vi "Begin.vi"(8 "error in (no error)":errorcluster, 11 "Catapult in":refnum<class "Catapult.lvclass">) -> (0 "error out":errorcluster, 3 "Catapult out":refnum<class "Catapult.lvclass">)   [LabVIEW 2013, in "Catapult.lvclass"]
uses:
  Catapult.lvclass
  <vilib>/Rock Robotics/WPI/CAN/Jaguar/SubVIs/WPI_CANJaguar_ControlMode.ctl
  <vilib>/Rock Robotics/SystemInterfaces/Typedef/FPGA_TypedefDigitalModule.ctl
  <vilib>/Rock Robotics/SystemInterfaces/DIO/FPGA_DIOChannel.ctl
  <vilib>/Rock Robotics/WPI/Solenoid/WPI_SolenoidChannel.ctl
  <vilib>/Rock Robotics/SystemInterfaces/Typedef/FPGA_TypedefSolenoidModule.ctl
  System/System.lvclass
  <vilib>/Rock Robotics/WPI/MotorControl/WPI_MotorControlOpenCANJaguar.vi
  <vilib>/Rock Robotics/WPI/Solenoid/WPI_SolenoidOpenSingle.vi
panel:
  in  "Solenoid Module (Module 1)":T1
  in  "Solenoid Channel":T2=enum."Solenoid 2"
  in  "DIO Channel":T3=enum."DIO 2"
  in  "Digital Module (Module 1)":T4
  in  "Catapult Control Mode":T5
  in  "Catapult Device Number":u8=8
  in  "Invert Catapult Motor":bool=TRUE
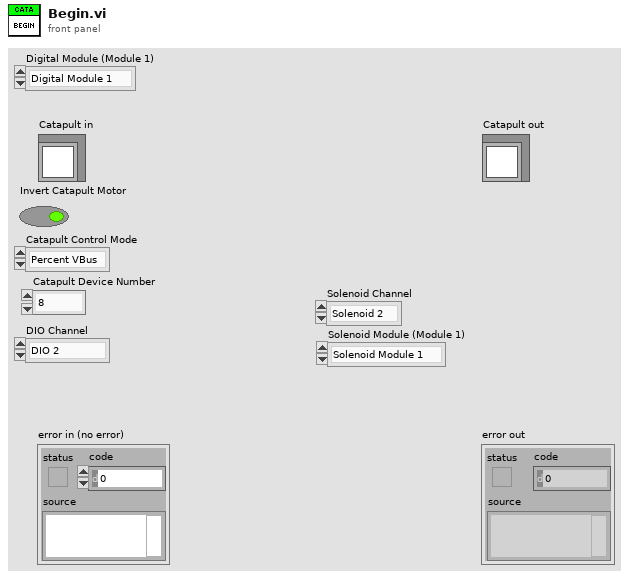
[diagram p1: front panel]
types:
  T1 = typedef "FPGA_TypedefSolenoidModule.ctl" = enum16{"Solenoid Module 1", "Solenoid Module 2"}
  T2 = typedef "WPI_SolenoidChannel.ctl" = enum8{"Solenoid 1", "Solenoid 2", "Solenoid 3", "Solenoid 4", "Solenoid 5", "Solenoid 6", "Solenoid 7", "Solenoid 8", "Invalid"}
  T3 = typedef "FPGA_DIOChannel.ctl" = enum8{"DIO 1", "DIO 2", "DIO 3", "DIO 4", "DIO 5", "DIO 6", "DIO 7", "DIO 8", "DIO 9", "DIO 10", "DIO 11", "DIO 12", "DIO 13", "DIO 14", "Invalid"}
  T4 = typedef "FPGA_TypedefDigitalModule.ctl" = enum16{"Digital Module 1", "Digital Module 2"}
  T5 = typedef "WPI_CANJaguar_ControlMode.ctl" = enum8{"Percent VBus", "Current", "Speed", "Position", "Voltage"}
  T6 = typedef "WPI_MotorControlDeviceRef.ctl" = cluster{"DeviceStatus":errorcluster, "Type":enum16{"PWM", "CAN"}, "PWM":cluster{"Digital Module":T4, "PWM Channel":T7, "DeadBand":T8}, "CAN":cluster{"Device Number":u8, "Control Mode":T5, "Semaphore":T9, "Max Vout":dbl}, "Invert":bool, "TransformRef":T10, "InvTransformRef":T10}
  T7 = typedef "FPGA_DIOPWMChannel.ctl" = enum8{"PWM 1", "PWM 2", "PWM 3", "PWM 4", "PWM 5", "PWM 6", "PWM 7", "PWM 8", "PWM 9", "PWM 10", "Invalid"}
  T8 = typedef "WPI_PWMDeadband.ctl" = cluster{"Name":string, "maxPositivePwm":i32, "minPositivePwm":i32, "centerPwm":i32, "maxNegativePwm":i32, "minNegativePwm":i32, "angularRange":u16}
  T9 = typedef "Semaphore RefNum" = refnum<k1>
  T10 = typedef "WPI_PWMTransform_ConPane.ctl" = refnum<vi>
  T11 = typedef "WPI_DigitalInputDevRef.ctl" = cluster{"DevStatus":errorcluster, "DIO Channel":T3, "Digital Module":T4}
  T12 = typedef "WPI_SolenoidDevRef.ctl" = cluster{"DevStatus":errorcluster, "Solenoid Module":T1, "Forward Solenoid Channel":T2, "Reverse Solenoid Channel":T2}
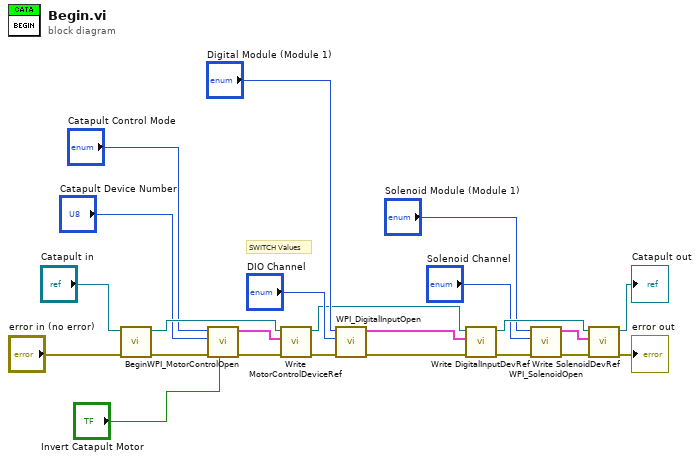
[diagram p0: block diagram]
diagram:
  # "SWITCH Values"
  n1 = call-parent "Begin.vi"("error in (no error)"="error in (no error)", "System in"="Catapult in") -> ("error out"=w20:errorcluster, "System out"=w21:refnum<class "Catapult.lvclass">)  [unwired: 8 in]
  n2 = call-poly <vilib>:"WPI_MotorControlOpen.vi"("Invert"="Invert Catapult Motor", "error in (no error)"=w20, "Device Number"="Catapult Device Number", "Control Mode"="Catapult Control Mode") -> ("error out"=w19:errorcluster, "MotorControlDeviceRef"=w15:T6)  [unwired: 6 in]
  n3 = call-dynamic "Write MotorControlDeviceRef.vi"("error in (no error)"=w19, "MotorControlDeviceRef"=w15, "Catapult in"=w21) -> ("error out"=w14:errorcluster, "Catapult out"=w9:refnum<class "Catapult.lvclass">)  [unwired: 7 in]
  n4 = call <vilib>:"WPI_DigitalInputOpen.vi"("error in (no error)"=w14, "DIO Channel"="DIO Channel", "Digital Module (Module 1)"="Digital Module (Module 1)") -> ("error out"=w13:errorcluster, "DigitalInputDevRef"=w12:T11)  [unwired: 7 in]
  n5 = call-dynamic "Write DigitalInputDevRef.vi"("error in (no error)"=w13, "DigitalInputDevRef"=w12, "Catapult in"=w9) -> ("error out"=w5:errorcluster, "Catapult out"=w8:refnum<class "Catapult.lvclass">)  [unwired: 7 in]
  n6 = call-poly <vilib>:"WPI_SolenoidOpen.vi"("error in (no error)"=w5, "Solenoid Channel"="Solenoid Channel", "Solenoid Module (Module 1)"="Solenoid Module (Module 1)") -> ("error out"=w4:errorcluster, "SolenoidDevRef"=w6:T12)  [unwired: 7 in]
  n7 = call-dynamic "Write SolenoidDevRef.vi"("error in (no error)"=w4, "SolenoidDevRef"=w6, "Catapult in"=w8) -> ("error out"=→"error out":errorcluster, "Catapult out"=→"Catapult out":refnum<class "Catapult.lvclass">)  [unwired: 7 in]
